vi "Generate Report as INI Section.vi"(7 "Parameters":variant, 8 "error in (no error)":errorcluster, 9 "Results":variant, 10 "Refnum in":T1, 11 "Analyze BaseClass in":refnum<class "Analyze BaseClass.lvclass">) -> (0 "error out":errorcluster, 2 "Refnum out":T1, 3 "Analyze BaseClass out":refnum<class "Analyze BaseClass.lvclass">)   [LabVIEW 2009, in "Analyze BaseClass.lvclass"]
uses:
  Analyze BaseClass.lvclass
  <vilib>/Utility/config.llb/Config Data RefNum.ctl
  <vilib>/Utility/config.llb/Write Key (I32).vi
  <vilib>/Utility/config.llb/NI_LVConfig.lvlib
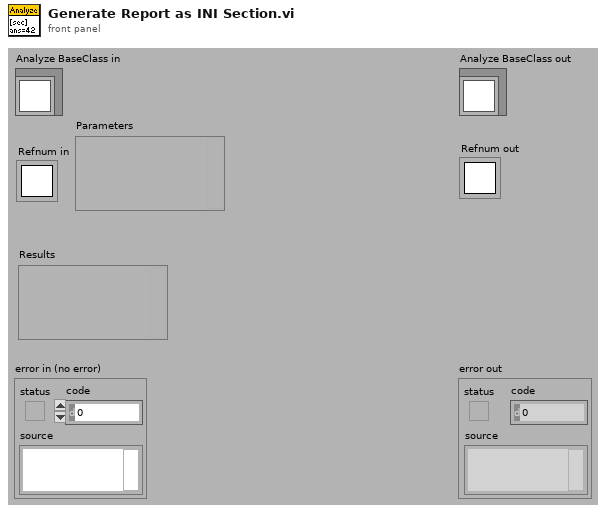
[diagram p1: front panel]
types:
  T1 = typedef "NI_LVConfig.lvlib/Config Data RefNum.ctl" = refnum<k1>
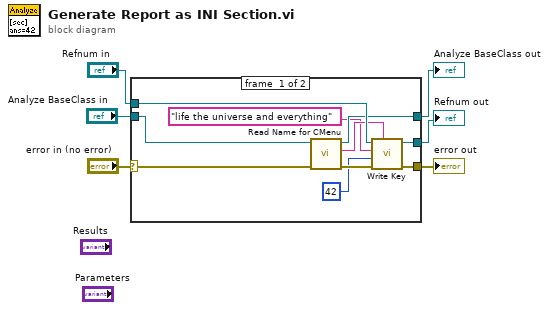
[diagram p0: block diagram]
diagram:
  n1 = case shown="No Error" "error in (no error)" {
    selector: "error in (no error)" -> [w16 w19]
    tunnel: [w12 w19] -> w5
    tunnel: [w10 w18] -> w3
    tunnel: "Analyze BaseClass in" -> [w11 w18]
    tunnel: [w14 w17] -> w2
    tunnel: "Refnum in" -> [w15 w17]
    frame #0 {
      n2 = call-dynamic "Read Name for CMenu.vi"("error in (no error)"=w16, "Analyze BaseClass in"=w11) -> ("error out"=w13:errorcluster, "Name for Context menu"=w9:string, "Analyze BaseClass out"=w10:refnum<class "Analyze BaseClass.lvclass">)  [unwired: 7 in]
      n3 = call-poly <vilib>:"Write Key.vi"("section"=w9, "error in (no error)"=w13, "value"=42, "key"="life the universe and everything", "refnum"=w15) -> ("error out"=w12:errorcluster, "refnum out"=w14:T1)  [unwired: 4 in, 1 out]
    }
    frame #1 {
    }
  }
  "error out" <- w5
  "Analyze BaseClass out" <- w3
  "Refnum out" <- w2
